vi "sub vi - Read Analog All v8.vi"() -> (2 "Analog loop time":dbl, 3 "array GRAPH":dynamicdata[](array[waveform]), 4 "LAB01":T2, 6 "LAB02":T3, 8 "LAB03":T4, 10 "LAB04":T5, 13 "deg C":dbl, 14 "array ERROR":errorcluster[](array[cluster]), 15 "LAB05":T6)   [LabVIEW 2013]
uses:
  <vilib>/addons/Electrical Power/Basic/Measurement/Power (1 Channel).vi
  <vilib>/addons/Electrical Power/Basic/Measurement/RMS (N Channels).vi
  <vilib>/addons/Electrical Power/Basic/Measurement/RMS (1 Channel).vi
  <vilib>/addons/Electrical Power/Basic/NI_EP_Basic.lvlib
panel:
  in  "Tab Control":T1(tab)
  out "LAB01-2 (PF)":dbl
  out "LAB01-1 (PF)":dbl
  out "LAB01-2 (V)":dbl
  out "LAB01-2 (A)":dbl
  out "LAB01-1 (V)":dbl
  out "LAB01-1 (A)":dbl
  out "LAB01-2 (GRAPH)":dynamicdata(graph)
  out "LAB01-1 (GRAPH)":dynamicdata(graph)
  out "LAB02-2 (PF)":dbl
  out "LAB02-1 (PF)":dbl
  out "LAB02-2 (V)":dbl
  out "LAB02-2 (A)":dbl
  out "LAB02-1 (V)":dbl
  out "LAB02-1 (A)":dbl
  out "LAB02-2 (GRAPH)":dynamicdata(graph)
  out "LAB02-1 (GRAPH)":dynamicdata(graph)
  out "LAB03-2 (PF)":dbl
  out "LAB03-1 (PF)":dbl
  out "LAB03-2 (V)":dbl
  out "LAB03-2 (A)":dbl
  out "LAB03-1 (V)":dbl
  out "LAB03-1 (A)":dbl
  out "LAB03-2 (GRAPH)":dynamicdata(graph)
  out "LAB03-1 (GRAPH)":dynamicdata(graph)
  out "LAB04-2 (PF)":dbl
  out "LAB04-1 (PF)":dbl
  out "LAB04-2 (V)":dbl
  out "LAB04-2 (A)":dbl
  out "LAB04-1 (V)":dbl
  out "LAB04-1 (A)":dbl
  out "LAB04-1 (GRAPH)":dynamicdata(graph)
  out "LAB04-2 (GRAPH)":dynamicdata(graph)
  out "LAB05-2 (PF)":dbl
  out "LAB05-1 (PF)":dbl
  out "LAB05-2 (V)":dbl
  out "LAB05-2 (A)":dbl
  out "LAB05-1 (V)":dbl
  out "LAB05-1 (A)":dbl
  out "LAB05-1 (GRAPH)":dynamicdata(graph)
  out "LAB05-2 (GRAPH)":dynamicdata(graph)
  out "A1 error":errorcluster
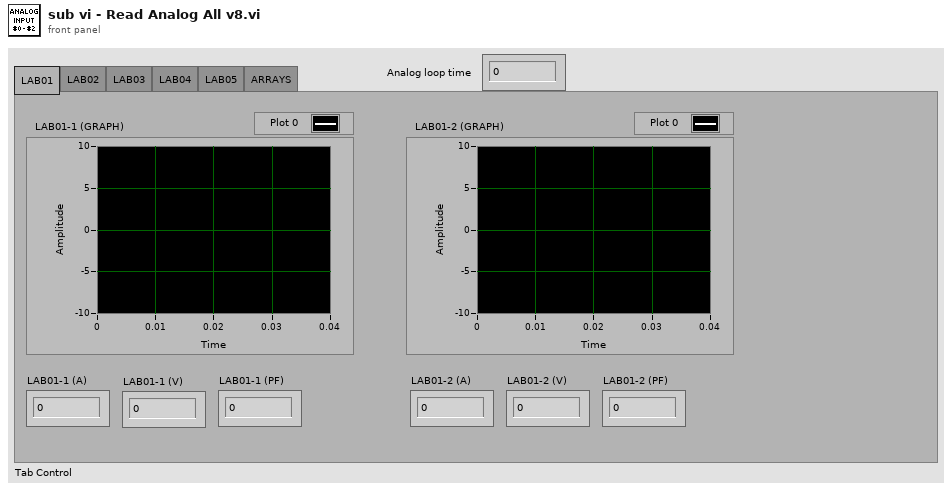
[diagram p1: front panel]
types:
  T1 = enum32{"LAB01", "LAB02", "LAB03", "LAB04", "LAB05", "ARRAYS"}
  T2 = cluster{"LAB01-1 (A)":dbl, "LAB01-1 (V)":dbl, "LAB01-1 (PF)":dbl, "LAB01-2 (A)":dbl, "LAB01-2 (V)":dbl, "LAB01-2 (PF)":dbl}
  T3 = cluster{"LAB02-1 (A)":dbl, "LAB02-1 (V)":dbl, "LAB02-1 (PF)":dbl, "LAB02-2 (A)":dbl, "LAB02-2 (V)":dbl, "LAB02-2 (PF)":dbl}
  T4 = cluster{"LAB03-1 (A)":dbl, "LAB03-1 (V)":dbl, "LAB03-1 (PF)":dbl, "LAB03-2 (A)":dbl, "LAB03-2 (V)":dbl, "LAB03-2 (PF)":dbl}
  T5 = cluster{"LAB04-1 (A)":dbl, "LAB04-1 (V)":dbl, "LAB04-1 (PF)":dbl, "LAB04-2 (A)":dbl, "LAB04-2 (V)":dbl, "LAB04-2 (PF)":dbl}
  T6 = cluster{"LAB05-1 (A)":dbl, "LAB05-1 (V)":dbl, "LAB05-1 (PF)":dbl, "LAB05-2 (A)":dbl, "LAB05-2 (V)":dbl, "LAB05-2 (PF)":dbl}
  T7 = typedef "NI_EP_Basic.lvlib/basic_Power Value.ctl" = cluster{"active power [W]":dbl, "apparent power [VA]":dbl, "reactive power [VAR]":dbl, "power factor":dbl}
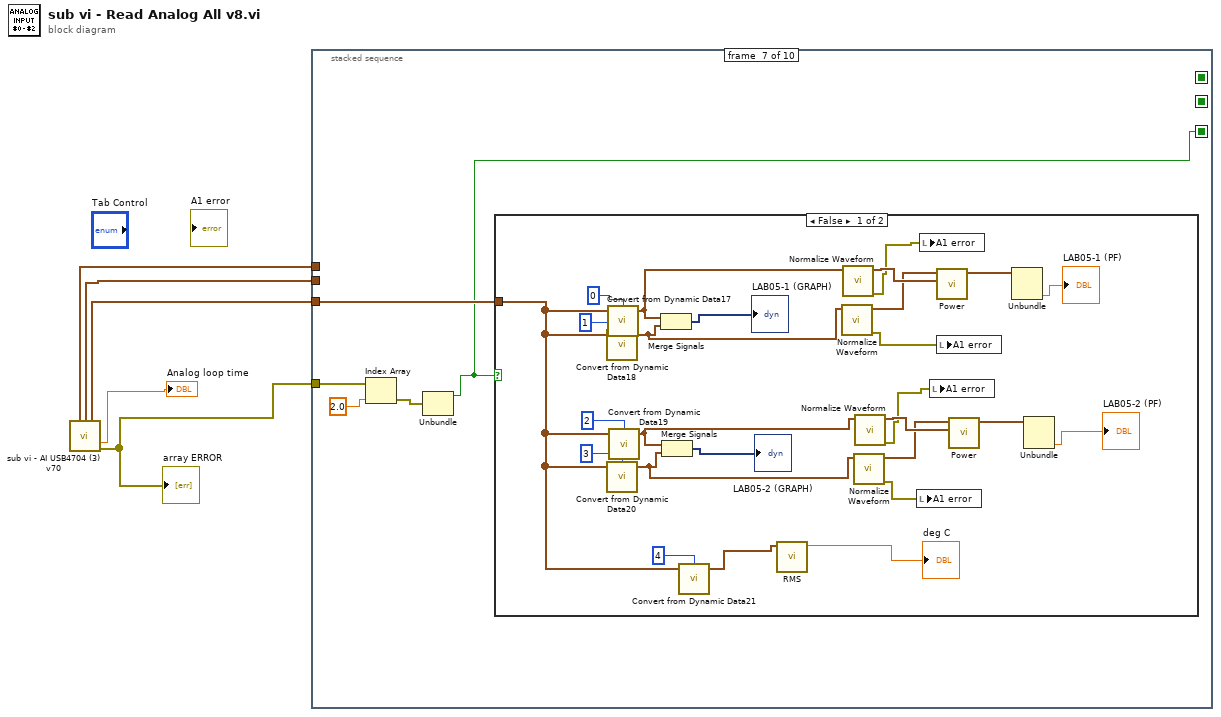
[diagram p0: block diagram]
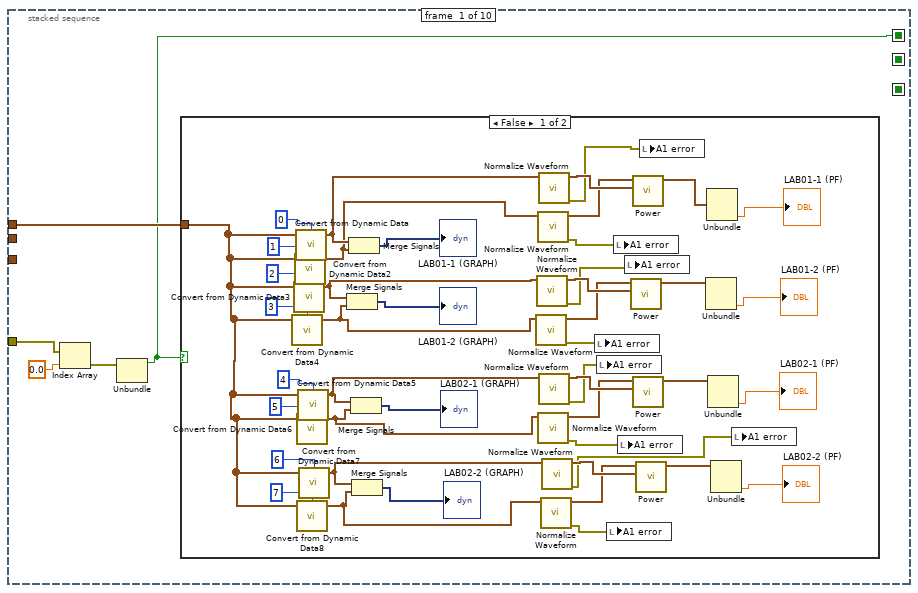
[diagram p2: hidden frame]
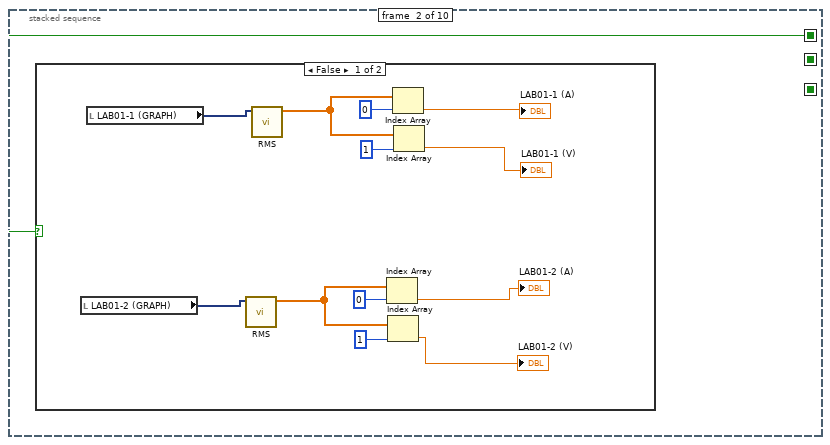
[diagram p4: hidden frame]
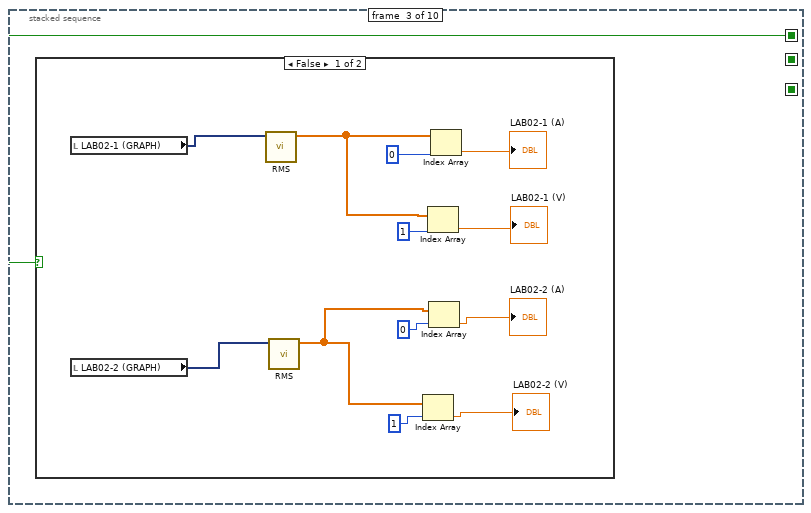
[diagram p6: hidden frame]
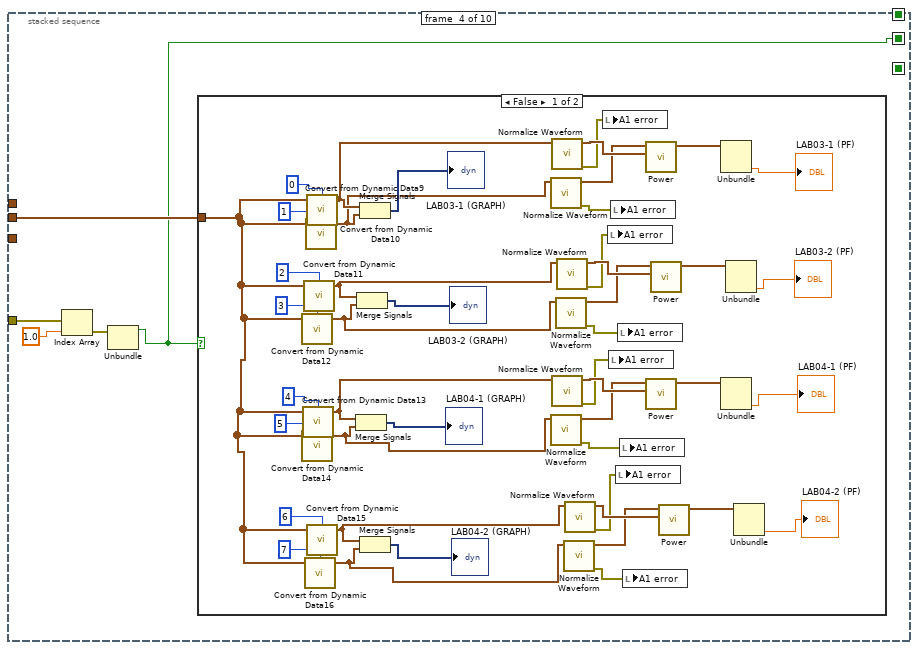
[diagram p8: hidden frame]
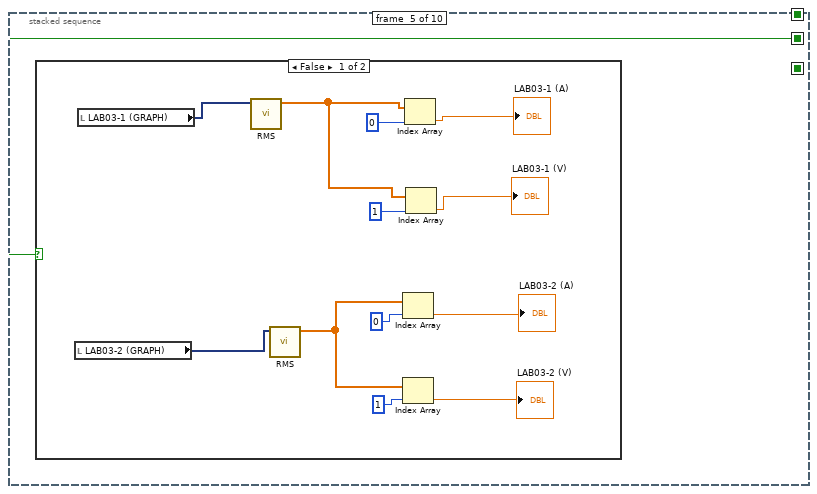
[diagram p10: hidden frame]
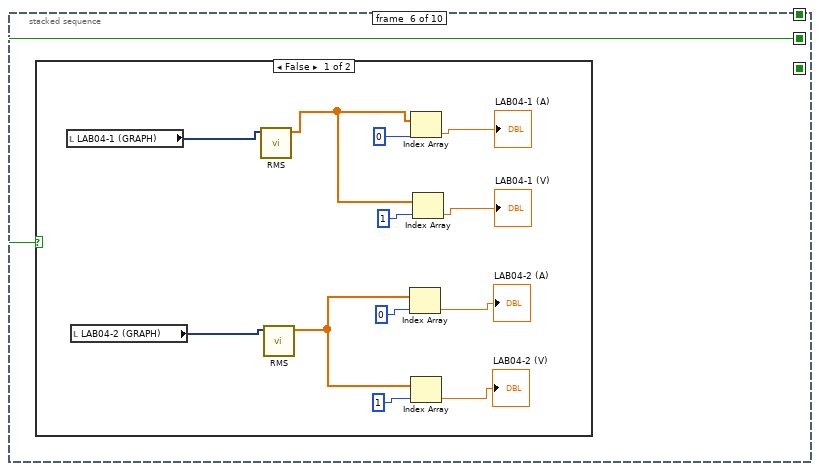
[diagram p12: hidden frame]
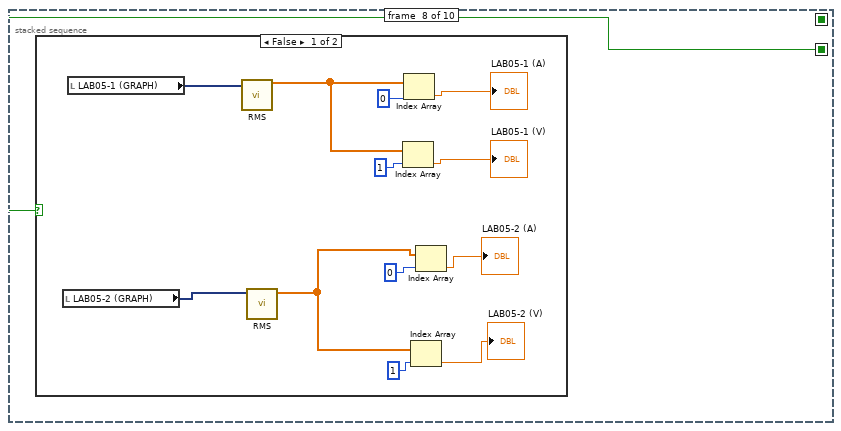
[diagram p15: hidden frame]
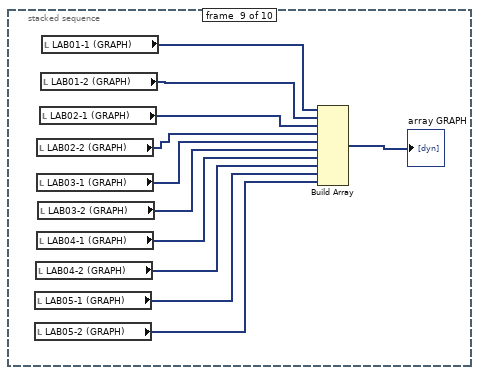
[diagram p17: hidden frame]
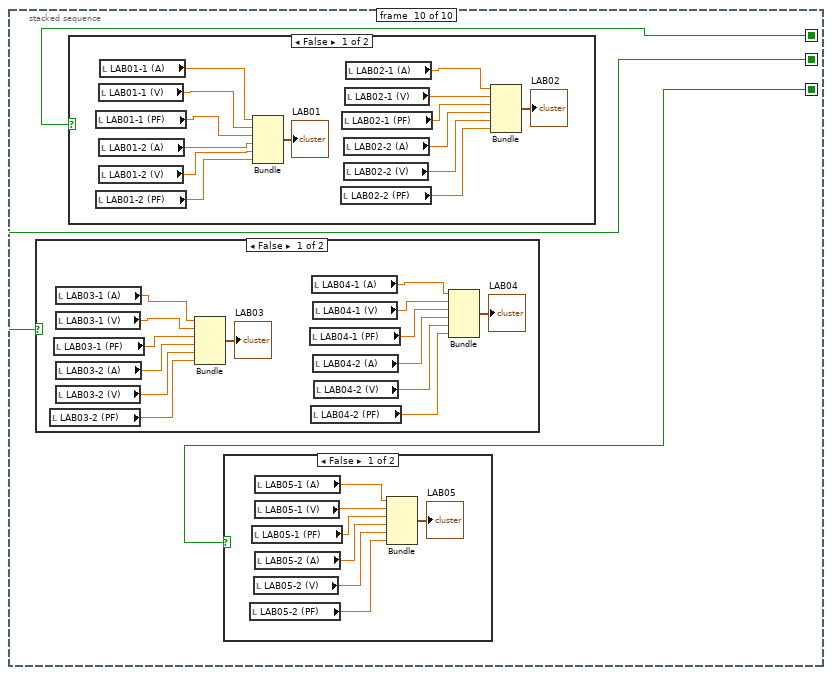
[diagram p18: hidden frame]
diagram:
  n1 = call "sub vi - AI USB4704 (3) v70.vi"() -> ("Graph 1"=w5:waveform(dbl)[], "Graph 2"=w4:waveform(dbl)[], "Graph 3"=w3:waveform(dbl)[], "loop time"=→"Analog loop time":dbl, "error array"=w1:errorcluster[])  [unwired: 11 in]
  "array ERROR" <- w1
  n2 = stacked-sequence {
    seq-local: [w6 _ _ _ _ _ _ _ _ _] -> [_ w56 w69 _ _ _ _ _ _ w215]
    seq-local: [_ _ _ w82 _ _ _ _ _ _] -> [_ _ _ _ w132 w145 _ _ _ w214]
    seq-local: [_ _ _ _ _ _ w158 _ _ _] -> [_ _ _ _ _ _ _ w189 _ w213]
    tunnel: w5 -> [w10 _ _ _ _ _ _ _ _ _]
    tunnel: w4 -> [_ _ _ w86 _ _ _ _ _ _]
    tunnel: w3 -> [_ _ _ _ _ _ w162 _ _ _]
    tunnel: w1 -> [w9 _ _ w85 _ _ w161 _ _ _]
    frame #0 {
      n3 = Index Array(array=w9, index=0.0) -> (element=w7:errorcluster)
      n4 = Unbundle(w7) -> ("status"=w6:bool)  [unwired: 2 out]
      n5 = case shown="False" w6 {
        tunnel: w10 -> [w45 _]
        frame False {
          n6 = call "Convert from Dynamic Data4"("Dynamic Data Type"=w45, "Channel"=3) -> ("Waveform"=w31:waveform(dbl))  [unwired: 2 in]
          n7 = call "Convert from Dynamic Data3"("Dynamic Data Type"=w45, "Channel"=2) -> ("Waveform"=w32:waveform(dbl))  [unwired: 2 in]
          n8 = call "Convert from Dynamic Data2"("Dynamic Data Type"=w45, "Channel"=1) -> ("Waveform"=w41:waveform(dbl))  [unwired: 2 in]
          n9 = call "Convert from Dynamic Data"("Dynamic Data Type"=w45, "Channel"=0) -> ("Waveform"=w42:waveform(dbl))  [unwired: 2 in]
          n10 = call "Convert from Dynamic Data6"("Dynamic Data Type"=w45, "Channel"=5) -> ("Waveform"=w26:waveform(dbl))  [unwired: 2 in]
          n11 = call "Convert from Dynamic Data8"("Dynamic Data Type"=w45, "Channel"=7) -> ("Waveform"=w20:waveform(dbl))  [unwired: 2 in]
          n12 = call "Convert from Dynamic Data5"("Dynamic Data Type"=w45, "Channel"=4) -> ("Waveform"=w27:waveform(dbl))  [unwired: 2 in]
          n13 = call "Convert from Dynamic Data7"("Dynamic Data Type"=w45, "Channel"=6) -> ("Waveform"=w21:waveform(dbl))  [unwired: 2 in]
          n14 = Merge Signals(w32, w31) -> (→"LAB01-2 (GRAPH)":dynamicdata)
          n15 = Merge Signals(w42, w41) -> (→"LAB01-1 (GRAPH)":dynamicdata)
          n16 = Merge Signals(w27, w26) -> (→"LAB02-1 (GRAPH)":dynamicdata)
          n17 = Merge Signals(w21, w20) -> (→"LAB02-2 (GRAPH)":dynamicdata)
          n18 = call <vilib>:"Normalize Waveform.vi"("waveform in"=w31) -> ("error out"=w15:errorcluster, "normalized waveform"=w35:waveform(dbl))  [unwired: 7 in, 2 out]
          n19 = call <vilib>:"Normalize Waveform.vi"("waveform in"=w32) -> ("error out"=w16:errorcluster, "normalized waveform"=w36:waveform(dbl))  [unwired: 7 in, 2 out]
          n20 = call <vilib>:"Normalize Waveform.vi"("waveform in"=w41) -> ("error out"=w17:errorcluster, "normalized waveform"=w39:waveform(dbl))  [unwired: 7 in, 2 out]
          n21 = call <vilib>:"Normalize Waveform.vi"("waveform in"=w26) -> ("error out"=w13:errorcluster, "normalized waveform"=w29:waveform(dbl))  [unwired: 7 in, 2 out]
          n22 = call <vilib>:"Normalize Waveform.vi"("waveform in"=w42) -> ("error out"=w18:errorcluster, "normalized waveform"=w40:waveform(dbl))  [unwired: 7 in, 2 out]
          n23 = call <vilib>:"Normalize Waveform.vi"("waveform in"=w27) -> ("error out"=w14:errorcluster, "normalized waveform"=w30:waveform(dbl))  [unwired: 7 in, 2 out]
          n24 = call <vilib>:"Normalize Waveform.vi"("waveform in"=w20) -> ("error out"=w11:errorcluster, "normalized waveform"=w23:waveform(dbl))  [unwired: 7 in, 2 out]
          n25 = call <vilib>:"Normalize Waveform.vi"("waveform in"=w21) -> ("error out"=w12:errorcluster, "normalized waveform"=w24:waveform(dbl))  [unwired: 7 in, 2 out]
          n26 = local write "A1 error"(w15) -> ()
          n27 = local write "A1 error"(w14) -> ()
          n28 = local write "A1 error"(w11) -> ()
          n29 = local write "A1 error"(w17) -> ()
          n30 = local write "A1 error"(w13) -> ()
          n31 = local write "A1 error"(w16) -> ()
          n32 = call-poly <vilib>:"Power.vi"("current waveform"=w36, "voltage waveform"=w35) -> ("power value"=w34:T7)  [unwired: 8 in, 1 out]
          n33 = call-poly <vilib>:"Power.vi"("current waveform"=w40, "voltage waveform"=w39) -> ("power value"=w38:T7)  [unwired: 8 in, 1 out]
          n34 = call-poly <vilib>:"Power.vi"("current waveform"=w30, "voltage waveform"=w29) -> ("power value"=w28:T7)  [unwired: 8 in, 1 out]
          n35 = call-poly <vilib>:"Power.vi"("current waveform"=w24, "voltage waveform"=w23) -> ("power value"=w22:T7)  [unwired: 8 in, 1 out]
          n36 = local write "A1 error"(w18) -> ()
          n37 = Unbundle(w34) -> ("power factor"=→"LAB01-2 (PF)":dbl)  [unwired: 3 out]
          n38 = Unbundle(w38) -> ("power factor"=→"LAB01-1 (PF)":dbl)  [unwired: 3 out]
          n39 = Unbundle(w28) -> ("power factor"=→"LAB02-1 (PF)":dbl)  [unwired: 3 out]
          n40 = Unbundle(w22) -> ("power factor"=→"LAB02-2 (PF)":dbl)  [unwired: 3 out]
          n41 = local write "A1 error"(w12) -> ()
        }
        frame True {
        }
      }
    }
    frame #1 {
      n42 = case shown="False" w56 {
        frame False {
          n43 = local read "LAB01-2 (GRAPH)"() -> (w65:dynamicdata)
          n44 = local read "LAB01-1 (GRAPH)"() -> (w59:dynamicdata)
          n45 = call-poly <vilib>:"RMS.vi"("waveforms"=w65) -> ("RMS values"=w64:dbl[])  [unwired: 9 in, 1 out]
          n46 = call-poly <vilib>:"RMS.vi"("waveforms"=w59) -> ("RMS values"=w68:dbl[])  [unwired: 9 in, 1 out]
          n47 = Index Array(array=w64, index=0) -> (element=→"LAB01-2 (A)":dbl)
          n48 = Index Array(array=w64, index=1) -> (element=→"LAB01-2 (V)":dbl)
          n49 = Index Array(array=w68, index=0) -> (element=→"LAB01-1 (A)":dbl)
          n50 = Index Array(array=w68, index=1) -> (element=→"LAB01-1 (V)":dbl)
        }
        frame True {
        }
      }
    }
    frame #2 {
      n51 = case shown="False" w69 {
        frame False {
          n52 = local read "LAB02-1 (GRAPH)"() -> (w77:dynamicdata)
          n53 = local read "LAB02-2 (GRAPH)"() -> (w73:dynamicdata)
          n54 = call-poly <vilib>:"RMS.vi"("waveforms"=w77) -> ("RMS values"=w76:dbl[])  [unwired: 9 in, 1 out]
          n55 = call-poly <vilib>:"RMS.vi"("waveforms"=w73) -> ("RMS values"=w72:dbl[])  [unwired: 9 in, 1 out]
          n56 = Index Array(array=w72, index=1) -> (element=→"LAB02-2 (V)":dbl)
          n57 = Index Array(array=w76, index=1) -> (element=→"LAB02-1 (V)":dbl)
          n58 = Index Array(array=w72, index=0) -> (element=→"LAB02-2 (A)":dbl)
          n59 = Index Array(array=w76, index=0) -> (element=→"LAB02-1 (A)":dbl)
        }
        frame True {
        }
      }
    }
    frame #3 {
      n60 = Index Array(array=w85, index=1.0) -> (element=w83:errorcluster)
      n61 = Unbundle(w83) -> ("status"=w82:bool)  [unwired: 2 out]
      n62 = case shown="False" w82 {
        tunnel: w86 -> [w119 _]
        frame False {
          n63 = call "Convert from Dynamic Data12"("Dynamic Data Type"=w119, "Channel"=3) -> ("Waveform"=w108:waveform(dbl))  [unwired: 2 in]
          n64 = call "Convert from Dynamic Data14"("Dynamic Data Type"=w119, "Channel"=5) -> ("Waveform"=w102:waveform(dbl))  [unwired: 2 in]
          n65 = call "Convert from Dynamic Data13"("Dynamic Data Type"=w119, "Channel"=4) -> ("Waveform"=w103:waveform(dbl))  [unwired: 2 in]
          n66 = call "Convert from Dynamic Data11"("Dynamic Data Type"=w119, "Channel"=2) -> ("Waveform"=w109:waveform(dbl))  [unwired: 2 in]
          n67 = call "Convert from Dynamic Data16"("Dynamic Data Type"=w119, "Channel"=7) -> ("Waveform"=w96:waveform(dbl))  [unwired: 2 in]
          n68 = call "Convert from Dynamic Data10"("Dynamic Data Type"=w119, "Channel"=1) -> ("Waveform"=w114:waveform(dbl))  [unwired: 2 in]
          n69 = call "Convert from Dynamic Data9"("Dynamic Data Type"=w119, "Channel"=0) -> ("Waveform"=w115:waveform(dbl))  [unwired: 2 in]
          n70 = call "Convert from Dynamic Data15"("Dynamic Data Type"=w119, "Channel"=6) -> ("Waveform"=w97:waveform(dbl))  [unwired: 2 in]
          n71 = Merge Signals(w103, w102) -> (→"LAB04-1 (GRAPH)":dynamicdata)
          n72 = Merge Signals(w109, w108) -> (→"LAB03-2 (GRAPH)":dynamicdata)
          n73 = Merge Signals(w115, w114) -> (→"LAB03-1 (GRAPH)":dynamicdata)
          n74 = Merge Signals(w97, w96) -> (→"LAB04-2 (GRAPH)":dynamicdata)
          n75 = call <vilib>:"Normalize Waveform.vi"("waveform in"=w114) -> ("error out"=w93:errorcluster, "normalized waveform"=w117:waveform(dbl))  [unwired: 7 in, 2 out]
          n76 = call <vilib>:"Normalize Waveform.vi"("waveform in"=w102) -> ("error out"=w89:errorcluster, "normalized waveform"=w105:waveform(dbl))  [unwired: 7 in, 2 out]
          n77 = call <vilib>:"Normalize Waveform.vi"("waveform in"=w115) -> ("error out"=w94:errorcluster, "normalized waveform"=w118:waveform(dbl))  [unwired: 7 in, 2 out]
          n78 = call <vilib>:"Normalize Waveform.vi"("waveform in"=w103) -> ("error out"=w90:errorcluster, "normalized waveform"=w106:waveform(dbl))  [unwired: 7 in, 2 out]
          n79 = call <vilib>:"Normalize Waveform.vi"("waveform in"=w108) -> ("error out"=w91:errorcluster, "normalized waveform"=w111:waveform(dbl))  [unwired: 7 in, 2 out]
          n80 = call <vilib>:"Normalize Waveform.vi"("waveform in"=w109) -> ("error out"=w92:errorcluster, "normalized waveform"=w112:waveform(dbl))  [unwired: 7 in, 2 out]
          n81 = call <vilib>:"Normalize Waveform.vi"("waveform in"=w96) -> ("error out"=w87:errorcluster, "normalized waveform"=w99:waveform(dbl))  [unwired: 7 in, 2 out]
          n82 = call <vilib>:"Normalize Waveform.vi"("waveform in"=w97) -> ("error out"=w88:errorcluster, "normalized waveform"=w100:waveform(dbl))  [unwired: 7 in, 2 out]
          n83 = local write "A1 error"(w94) -> ()
          n84 = local write "A1 error"(w92) -> ()
          n85 = local write "A1 error"(w90) -> ()
          n86 = local write "A1 error"(w93) -> ()
          n87 = local write "A1 error"(w88) -> ()
          n88 = local write "A1 error"(w91) -> ()
          n89 = local write "A1 error"(w89) -> ()
          n90 = local write "A1 error"(w87) -> ()
          n91 = call-poly <vilib>:"Power.vi"("current waveform"=w118, "voltage waveform"=w117) -> ("power value"=w116:T7)  [unwired: 8 in, 1 out]
          n92 = call-poly <vilib>:"Power.vi"("current waveform"=w106, "voltage waveform"=w105) -> ("power value"=w104:T7)  [unwired: 8 in, 1 out]
          n93 = call-poly <vilib>:"Power.vi"("current waveform"=w112, "voltage waveform"=w111) -> ("power value"=w110:T7)  [unwired: 8 in, 1 out]
          n94 = call-poly <vilib>:"Power.vi"("current waveform"=w100, "voltage waveform"=w99) -> ("power value"=w98:T7)  [unwired: 8 in, 1 out]
          n95 = Unbundle(w116) -> ("power factor"=→"LAB03-1 (PF)":dbl)  [unwired: 3 out]
          n96 = Unbundle(w104) -> ("power factor"=→"LAB04-1 (PF)":dbl)  [unwired: 3 out]
          n97 = Unbundle(w110) -> ("power factor"=→"LAB03-2 (PF)":dbl)  [unwired: 3 out]
          n98 = Unbundle(w98) -> ("power factor"=→"LAB04-2 (PF)":dbl)  [unwired: 3 out]
        }
        frame True {
        }
      }
    }
    frame #4 {
      n99 = case shown="False" w132 {
        frame False {
          n100 = local read "LAB03-2 (GRAPH)"() -> (w139:dynamicdata)
          n101 = local read "LAB03-1 (GRAPH)"() -> (w140:dynamicdata)
          n102 = call-poly <vilib>:"RMS.vi"("waveforms"=w140) -> ("RMS values"=w138:dbl[])  [unwired: 9 in, 1 out]
          n103 = call-poly <vilib>:"RMS.vi"("waveforms"=w139) -> ("RMS values"=w135:dbl[])  [unwired: 9 in, 1 out]
          n104 = Index Array(array=w135, index=0) -> (element=→"LAB03-2 (A)":dbl)
          n105 = Index Array(array=w135, index=1) -> (element=→"LAB03-2 (V)":dbl)
          n106 = Index Array(array=w138, index=0) -> (element=→"LAB03-1 (A)":dbl)
          n107 = Index Array(array=w138, index=1) -> (element=→"LAB03-1 (V)":dbl)
        }
        frame True {
        }
      }
    }
    frame #5 {
      n108 = case shown="False" w145 {
        frame False {
          n109 = local read "LAB04-1 (GRAPH)"() -> (w153:dynamicdata)
          n110 = local read "LAB04-2 (GRAPH)"() -> (w149:dynamicdata)
          n111 = call-poly <vilib>:"RMS.vi"("waveforms"=w153) -> ("RMS values"=w152:dbl[])  [unwired: 9 in, 1 out]
          n112 = call-poly <vilib>:"RMS.vi"("waveforms"=w149) -> ("RMS values"=w148:dbl[])  [unwired: 9 in, 1 out]
          n113 = Index Array(array=w148, index=0) -> (element=→"LAB04-2 (A)":dbl)
          n114 = Index Array(array=w152, index=0) -> (element=→"LAB04-1 (A)":dbl)
          n115 = Index Array(array=w148, index=1) -> (element=→"LAB04-2 (V)":dbl)
          n116 = Index Array(array=w152, index=1) -> (element=→"LAB04-1 (V)":dbl)
        }
        frame True {
        }
      }
    }
    frame #6 {
      n117 = Index Array(array=w161, index=2.0) -> (element=w159:errorcluster)
      n118 = Unbundle(w159) -> ("status"=w158:bool)  [unwired: 2 out]
      n119 = case shown="False" w158 {
        tunnel: w162 -> [w165 _]
        frame False {
          n120 = call "Convert from Dynamic Data18"("Dynamic Data Type"=w165, "Channel"=1) -> ("Waveform"=w178:waveform(dbl))  [unwired: 2 in]
          n121 = call "Convert from Dynamic Data20"("Dynamic Data Type"=w165, "Channel"=3) -> ("Waveform"=w172:waveform(dbl))  [unwired: 2 in]
          n122 = call "Convert from Dynamic Data17"("Dynamic Data Type"=w165, "Channel"=0) -> ("Waveform"=w179:waveform(dbl))  [unwired: 2 in]
          n123 = call "Convert from Dynamic Data19"("Dynamic Data Type"=w165, "Channel"=2) -> ("Waveform"=w173:waveform(dbl))  [unwired: 2 in]
          n124 = Merge Signals(w179, w178) -> (→"LAB05-1 (GRAPH)":dynamicdata)
          n125 = Merge Signals(w173, w172) -> (→"LAB05-2 (GRAPH)":dynamicdata)
          n126 = call "Convert from Dynamic Data21"("Dynamic Data Type"=w165, "Channel"=4) -> ("Waveform"=w164:waveform(dbl))  [unwired: 2 in]
          n127 = call-poly <vilib>:"RMS.vi"("waveform"=w164) -> ("RMS value"=→"deg C":dbl)  [unwired: 9 in, 1 out]
          n128 = call <vilib>:"Normalize Waveform.vi"("waveform in"=w178) -> ("error out"=w170:errorcluster, "normalized waveform"=w181:waveform(dbl))  [unwired: 7 in, 2 out]
          n129 = call <vilib>:"Normalize Waveform.vi"("waveform in"=w179) -> ("error out"=w169:errorcluster, "normalized waveform"=w182:waveform(dbl))  [unwired: 7 in, 2 out]
          n130 = call <vilib>:"Normalize Waveform.vi"("waveform in"=w172) -> ("error out"=w168:errorcluster, "normalized waveform"=w175:waveform(dbl))  [unwired: 7 in, 2 out]
          n131 = call <vilib>:"Normalize Waveform.vi"("waveform in"=w173) -> ("error out"=w167:errorcluster, "normalized waveform"=w176:waveform(dbl))  [unwired: 7 in, 2 out]
          n132 = local write "A1 error"(w168) -> ()
          n133 = local write "A1 error"(w169) -> ()
          n134 = local write "A1 error"(w167) -> ()
          n135 = call-poly <vilib>:"Power.vi"("current waveform"=w182, "voltage waveform"=w181) -> ("power value"=w180:T7)  [unwired: 8 in, 1 out]
          n136 = local write "A1 error"(w170) -> ()
          n137 = call-poly <vilib>:"Power.vi"("current waveform"=w176, "voltage waveform"=w175) -> ("power value"=w174:T7)  [unwired: 8 in, 1 out]
          n138 = Unbundle(w180) -> ("power factor"=→"LAB05-1 (PF)":dbl)  [unwired: 3 out]
          n139 = Unbundle(w174) -> ("power factor"=→"LAB05-2 (PF)":dbl)  [unwired: 3 out]
        }
        frame True {
        }
      }
    }
    frame #7 {
      n140 = case shown="False" w189 {
        frame False {
          n141 = local read "LAB05-2 (GRAPH)"() -> (w196:dynamicdata)
          n142 = local read "LAB05-1 (GRAPH)"() -> (w197:dynamicdata)
          n143 = call-poly <vilib>:"RMS.vi"("waveforms"=w197) -> ("RMS values"=w195:dbl[])  [unwired: 9 in, 1 out]
          n144 = call-poly <vilib>:"RMS.vi"("waveforms"=w196) -> ("RMS values"=w194:dbl[])  [unwired: 9 in, 1 out]
          n145 = Index Array(array=w195, index=1) -> (element=→"LAB05-1 (V)":dbl)
          n146 = Index Array(array=w195, index=0) -> (element=→"LAB05-1 (A)":dbl)
          n147 = Index Array(array=w194, index=1) -> (element=→"LAB05-2 (V)":dbl)
          n148 = Index Array(array=w194, index=0) -> (element=→"LAB05-2 (A)":dbl)
        }
        frame True {
        }
      }
    }
    frame #8 {
      n149 = local read "LAB05-1 (GRAPH)"() -> (w204:dynamicdata)
      n150 = local read "LAB05-2 (GRAPH)"() -> (w203:dynamicdata)
      n151 = local read "LAB04-2 (GRAPH)"() -> (w205:dynamicdata)
      n152 = local read "LAB02-2 (GRAPH)"() -> (w209:dynamicdata)
      n153 = local read "LAB03-1 (GRAPH)"() -> (w208:dynamicdata)
      n154 = local read "LAB04-1 (GRAPH)"() -> (w206:dynamicdata)
      n155 = local read "LAB03-2 (GRAPH)"() -> (w207:dynamicdata)
      n156 = local read "LAB02-1 (GRAPH)"() -> (w210:dynamicdata)
      n157 = local read "LAB01-2 (GRAPH)"() -> (w211:dynamicdata)
      n158 = local read "LAB01-1 (GRAPH)"() -> (w212:dynamicdata)
      n159 = Build Array(w212, w211, w210, w209, w208, w207, w206, w205, w204, w203) -> (→"array GRAPH":dynamicdata[])
    }
    frame #9 {
      n160 = case shown="False" w214 {
        frame False {
          n161 = local read "LAB03-2 (PF)"() -> (w231:dbl)
          n162 = local read "LAB03-1 (PF)"() -> (w234:dbl)
          n163 = local read "LAB03-1 (A)"() -> (w236:dbl)
          n164 = local read "LAB03-1 (V)"() -> (w235:dbl)
          n165 = local read "LAB03-2 (A)"() -> (w233:dbl)
          n166 = local read "LAB03-2 (V)"() -> (w232:dbl)
          n167 = Bundle("LAB03-1 (A)"=w236, "LAB03-1 (V)"=w235, "LAB03-1 (PF)"=w234, "LAB03-2 (A)"=w233, "LAB03-2 (V)"=w232, "LAB03-2 (PF)"=w231) -> (→"LAB03":T4)  [unwired: 1 in]
          n168 = local read "LAB04-1 (PF)"() -> (w228:dbl)
          n169 = local read "LAB04-2 (PF)"() -> (w225:dbl)
          n170 = local read "LAB04-1 (A)"() -> (w230:dbl)
          n171 = local read "LAB04-1 (V)"() -> (w229:dbl)
          n172 = local read "LAB04-2 (A)"() -> (w227:dbl)
          n173 = local read "LAB04-2 (V)"() -> (w226:dbl)
          n174 = Bundle("LAB04-1 (A)"=w230, "LAB04-1 (V)"=w229, "LAB04-1 (PF)"=w228, "LAB04-2 (A)"=w227, "LAB04-2 (V)"=w226, "LAB04-2 (PF)"=w225) -> (→"LAB04":T5)  [unwired: 1 in]
        }
        frame True {
        }
      }
      n175 = case shown="False" w215 {
        frame False {
          n176 = local read "LAB01-1 (PF)"() -> (w241:dbl)
          n177 = local read "LAB01-2 (PF)"() -> (w238:dbl)
          n178 = local read "LAB01-1 (V)"() -> (w242:dbl)
          n179 = local read "LAB01-2 (A)"() -> (w240:dbl)
          n180 = local read "LAB01-2 (V)"() -> (w239:dbl)
          n181 = local read "LAB01-1 (A)"() -> (w243:dbl)
          n182 = Bundle("LAB01-1 (A)"=w243, "LAB01-1 (V)"=w242, "LAB01-1 (PF)"=w241, "LAB01-2 (A)"=w240, "LAB01-2 (V)"=w239, "LAB01-2 (PF)"=w238) -> (→"LAB01":T2)  [unwired: 1 in]
          n183 = local read "LAB02-2 (PF)"() -> (w245:dbl)
          n184 = local read "LAB02-1 (PF)"() -> (w248:dbl)
          n185 = local read "LAB02-2 (A)"() -> (w247:dbl)
          n186 = local read "LAB02-2 (V)"() -> (w246:dbl)
          n187 = local read "LAB02-1 (V)"() -> (w249:dbl)
          n188 = local read "LAB02-1 (A)"() -> (w250:dbl)
          n189 = Bundle("LAB02-1 (A)"=w250, "LAB02-1 (V)"=w249, "LAB02-1 (PF)"=w248, "LAB02-2 (A)"=w247, "LAB02-2 (V)"=w246, "LAB02-2 (PF)"=w245) -> (→"LAB02":T3)  [unwired: 1 in]
        }
        frame True {
        }
      }
      n190 = case shown="False" w213 {
        frame False {
          n191 = local read "LAB05-2 (PF)"() -> (w217:dbl)
          n192 = local read "LAB05-1 (PF)"() -> (w220:dbl)
          n193 = local read "LAB05-2 (V)"() -> (w218:dbl)
          n194 = local read "LAB05-1 (A)"() -> (w222:dbl)
          n195 = local read "LAB05-1 (V)"() -> (w221:dbl)
          n196 = local read "LAB05-2 (A)"() -> (w219:dbl)
          n197 = Bundle("LAB05-1 (A)"=w222, "LAB05-1 (V)"=w221, "LAB05-1 (PF)"=w220, "LAB05-2 (A)"=w219, "LAB05-2 (V)"=w218, "LAB05-2 (PF)"=w217) -> (→"LAB05":T6)  [unwired: 1 in]
        }
        frame True {
        }
      }
    }
  }
